vi "Create Test Projects.vi"(4 "error in":errorcluster) -> (0 "error out":errorcluster)   [LabVIEW 2025]
doc: "This VI creates all configured test projects for unit testing. The configuration file <i>Test Project Definition.xml</i> must lie in the same folder as this VI."
uses:
  Project Definition--cluster.ctl
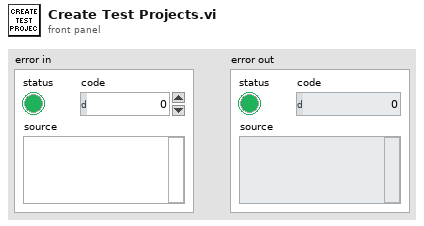
[diagram p1: front panel]
types:
  T1 = typedef "Project Definition--cluster.ctl" = cluster{"Name":string, "Description":string, "Elements":path[]}
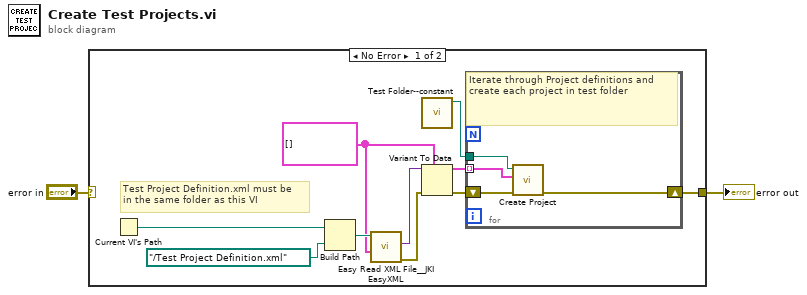
[diagram p0: block diagram]
diagram:
  n1 = case shown="No Error" "error in" {
    selector: "error in" -> [_ w17]
    tunnel: [w9 w17] -> w1
    frame No Error {
      w5 = T1[] [] ("Array")
      # "Test Project Definition.xml must be\nin the same folder as this VI"
      n2 = Current VI's Path() -> (path=w12:path)
      n3 = Build Path(base path=w12, name or relative path=path "../Test Project Definition.xml") -> (appended path=w6:path)
      n4 = call <vilib>:"Easy Read XML File__JKI EasyXML.vi"("LabVIEW Data (Type)"=w5, "XML File Path"=w6) -> ("error out"=w3:errorcluster, "LabVIEW Data"=w4:variant)  [unwired: 7 in, 1 out]
      n5 = call "Test Folder--constant.vi"() -> ("Test Folder"=w8:path)  [unwired: 7 in]
      n6 = Variant To Data(error in=w3, type=w5, Variant=w4) -> (data=w7:T1[], error out=w10:errorcluster)
      n7 = for {
        tunnel: w8 -> [w16]
        tunnel: w7 -> [w15] mode=indexing
        shift-right: [w13] -> w9
        shift-left: w10 -> [w14]
        # "Iterate through Project definitions and create each project in test folder"
        n8 = call "Create Project.vi"("error in"=w14, "Project Definition"=w15, "Path"=w16) -> ("error out"=w13:errorcluster)  [unwired: 4 in]
      }
    }
    frame Error {
      # "Pass error without further action"
    }
  }
  "error out" <- w1
